vi "ProcessName.vi"() -> (1 "process name":string)   [LabVIEW 2017, in "TracePointDisplay.lvlib"]
uses:
  <vilib>/addons/InsightCM/Devices/Shared/Common/TracePointDisplay/TracePointDisplay.lvlib
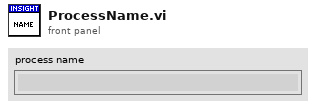
[diagram p1: front panel]
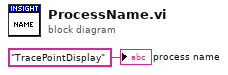
[diagram p0: block diagram]
diagram:
  "process name" <- "TracePointDisplay" ("ProcessName")
